vi "task1.vi"() -> ()   [LabVIEW 2021]
panel:
  out "Array":dbl[](array[numeric])
  in  "Numeric":i32
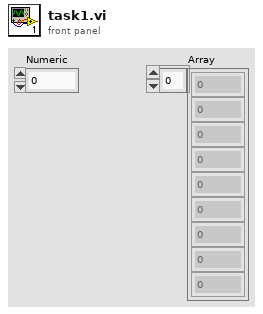
[diagram p1: front panel]
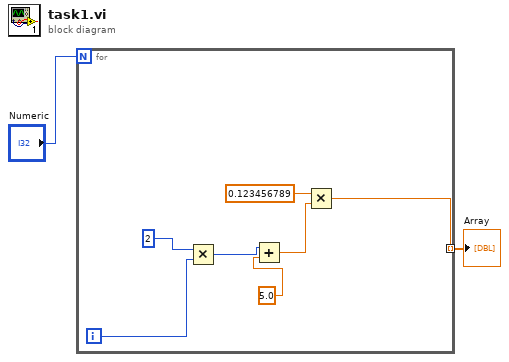
[diagram p0: block diagram]
diagram:
  n1 = for {
    N: "Numeric" -> [_]
    tunnel: [w3] -> w1 mode=indexing
    i -> [w8]
    n2 = Multiply(x=2, y=w8) -> (x*y=w6:i32)
    n3 = Add(x=w6, y=5.0 ("x*y")) -> (x+y=w4:dbl)
    n4 = Multiply(x=0.123456789, y=w4) -> (x*y=w3:dbl)
  }
  "Array" <- w1
